vi "Re_run_Gnuplot.vi"(0 "Plot folder (dialog if empty)":path) -> ()   [LabVIEW 2014]
panel:
  in  "Data file":string
  in  "stop":bool
  in  "OK Button":bool
  in  "Gnuplot script file":string
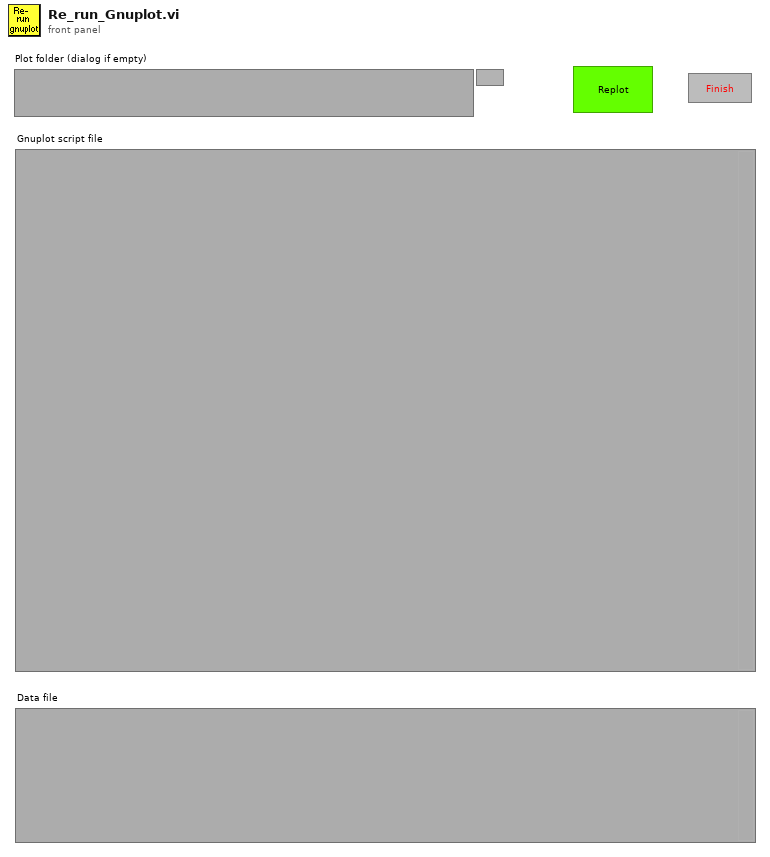
[diagram p1: front panel]
types:
  T1 = enum32{"existing file", "new file", "new or existing file", "existing dir", "new dir", "new or existing dir", "existing file (use LLBs)", "new file (use LLBs)", "new or existing file (use LLBs)", "new or existing file or directory (use LLBs)"}
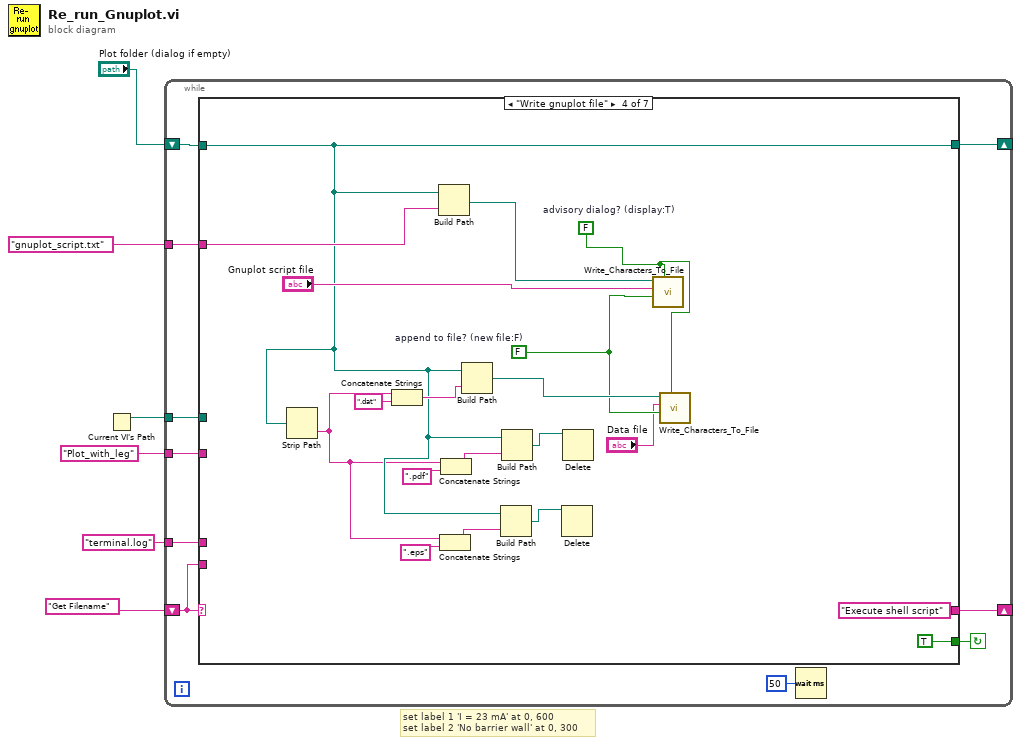
[diagram p0: block diagram]
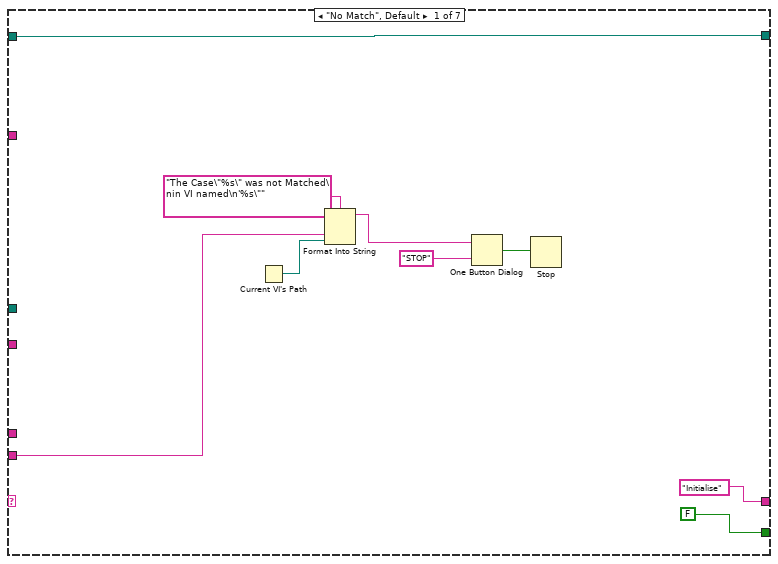
[diagram p2: hidden frame]
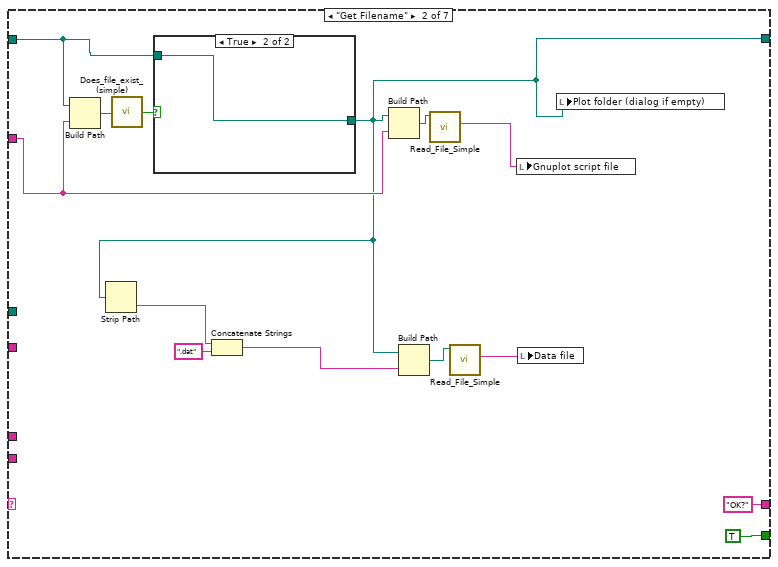
[diagram p3: hidden frame]
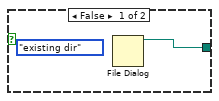
[diagram p4: hidden frame]
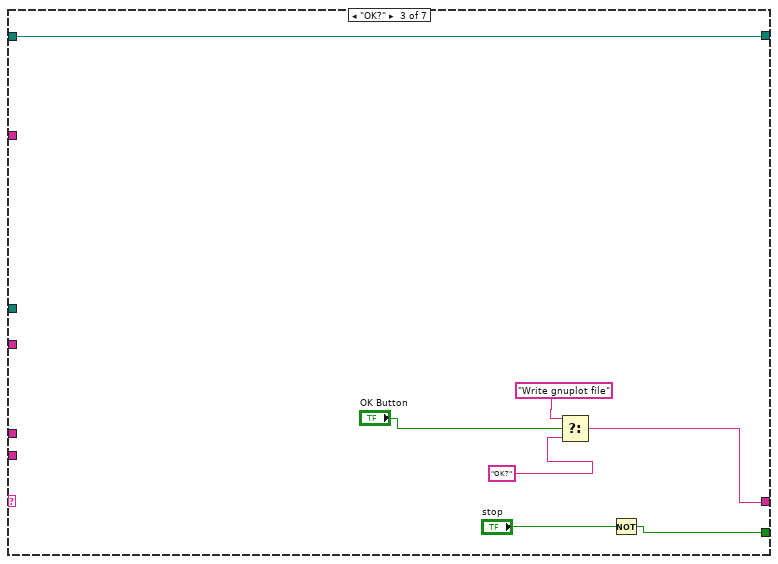
[diagram p5: hidden frame]
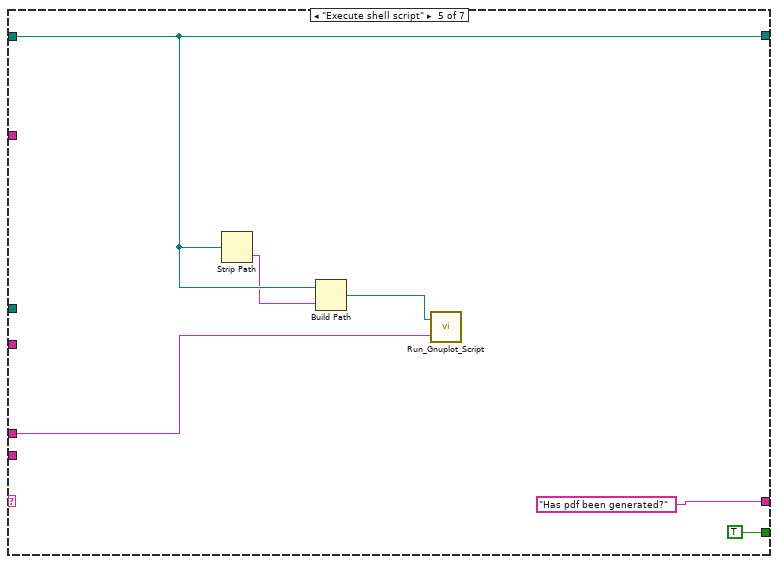
[diagram p6: hidden frame]
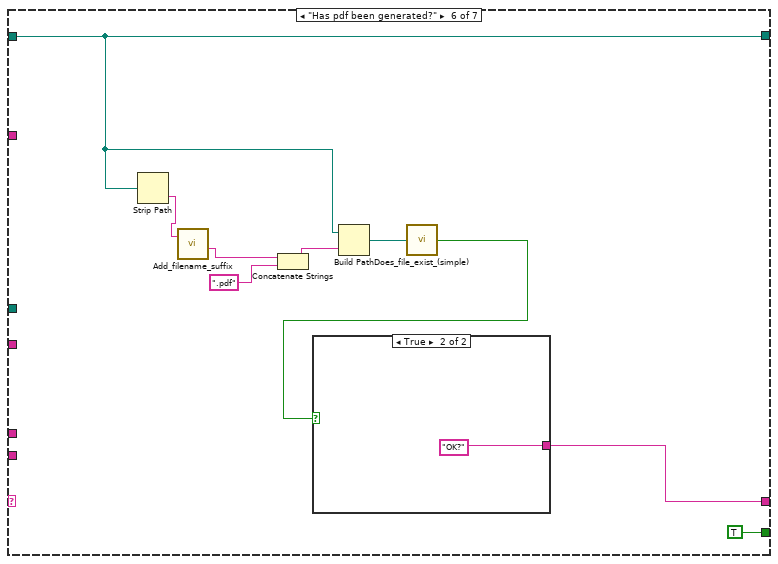
[diagram p7: hidden frame]
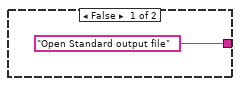
[diagram p8: hidden frame]
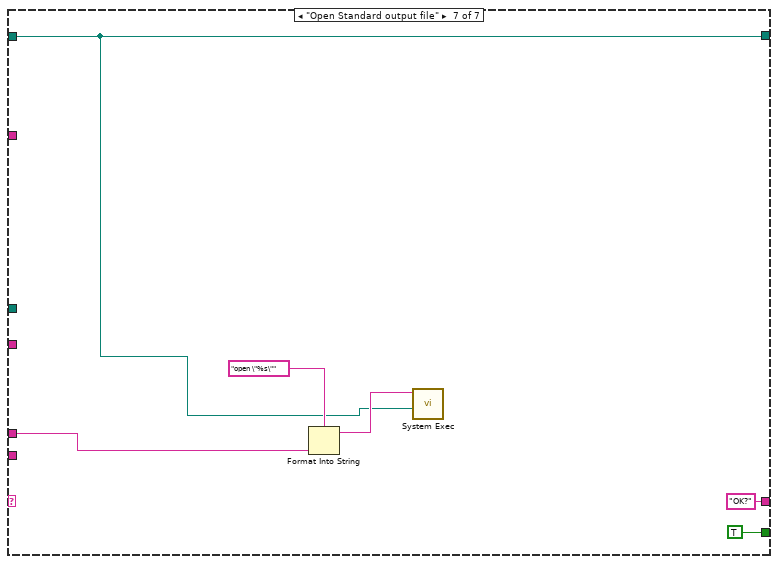
[diagram p9: hidden frame]
diagram:
  # "set label 1 'I = 23 mA' at 0, 600\nset label 2 'No barrier wall' at 0, 300"
  n1 = Current VI's Path() -> (path=w5:path)
  n2 = while {
    shift-left: "Get Filename" -> [w14]
    shift-right: [w15] -> _
    tunnel: w5 -> [w13]
    shift-right: [w12] -> _
    shift-left: "Plot folder (dialog if empty)" -> [w11]
    tunnel: "Plot_with_leg" ("name or relative path") -> [w10]
    tunnel: "terminal.log" -> [w9]
    tunnel: "gnuplot_script.txt" -> [w8]
    stop <- w16 continue-if-true
    n3 = case shown="\"Write gnuplot file\"" w14 {
      tunnel: [FALSE TRUE ("Top Level") w42 TRUE ("Top Level") TRUE ("Top Level") TRUE ("Top Level") TRUE ("Top Level")] -> w16
      tunnel: ["Initialise" "OK?" ("t") w48 "Execute shell script" ("t") "Has pdf been generated?" ("t") w79 "OK?" ("t")] -> w15
      tunnel: w14 -> [w20 _ _ _ _ _ _]
      tunnel: w13 -> [_ _ _ _ _ _ _]
      tunnel: [w17 w31 w45 w50 w70 w74 w85] -> w12
      tunnel: w11 -> [w17 w35 w45 w50 w70 w74 w85]
      tunnel: w10 -> [_ _ _ _ _ _ _]
      tunnel: w9 -> [_ _ _ _ w71 _ w87]
      tunnel: w8 -> [_ w34 _ w63 _ _ _]
      frame "No Match", Default {
        n4 = Current VI's Path() -> (path=w19:path)
        n5 = Format Into String(format string="The Case\"%s\" was not Matched\nin VI named\n'%s\"" ("Format String"), w20, w19) -> (resulting string=w23:string)  [unwired: 2 in, 1 out]
        n6 = One Button Dialog(message=w23, button name ("OK")="STOP") -> (true=w21:bool)
        n7 = Stop(stop? (T)=w21) -> ()
      }
      frame "Get Filename" {
        n8 = Build Path(base path=w35, name or relative path=w34) -> (appended path=w33:path)
        n9 = call "Does_file_exist_(simple).vi"("Pathname"=w33) -> ("exists?"=w32:bool)
        n10 = case shown="True" w32 {
          tunnel: [w40 w41] -> w31
          tunnel: w35 -> [_ w41]
          frame False {
            (unwired) T1."existing dir" ("select mode (2)")
            n11 = File Dialog() -> (3:w40:path)  [unwired: 1 in, 9 out]
          }
          frame True {
          }
        }
        n12 = Strip Path(path=w31) -> (name=w30:string)  [unwired: 1 out]
        n13 = Concatenate Strings(w30, ".dat" ("string")) -> (w28:string)
        n14 = Build Path(base path=w31, name or relative path=w34) -> (appended path=w36:path)
        n15 = Build Path(base path=w31, name or relative path=w28) -> (appended path=w27:path)
        n16 = call "Read_File_Simple.vi"("Filename"=w36) -> ("string"=w38:string)  [unwired: 2 in, 7 out]
        n17 = call "Read_File_Simple.vi"("Filename"=w27) -> ("string"=w26:string)  [unwired: 2 in, 7 out]
        n18 = local write "Gnuplot script file"(w38) -> ()
        n19 = local write "Data file"(w26) -> ()
        n20 = local write "Plot folder (dialog if empty)"(w31) -> ()
      }
      frame "OK?" {
        n21 = Select(t="Write gnuplot file", s="OK Button", f="OK?") -> (s? t:f=w48:string)
        n22 = Not(x="stop") -> (.not. x?=w42:bool)
      }
      frame "Write gnuplot file" {
        w59 = FALSE  # append to file? (new file:F)
        w58 = FALSE  # advisory dialog? (display:T)
        n23 = Strip Path(path=w50) -> (name=w49:string)  [unwired: 1 out]
        n24 = Concatenate Strings(w49, ".dat" ("string")) -> (w61:string)
        n25 = Build Path(base path=w50, name or relative path=w63) -> (appended path=w67:path)
        n26 = Concatenate Strings(w49, ".eps" ("string")) -> (w51:string)
        n27 = Concatenate Strings(w49, ".pdf" ("string")) -> (w56:string)
        n28 = Build Path(base path=w50, name or relative path=w61) -> (appended path=w60:path)
        n29 = Build Path(base path=w50, name or relative path=w51) -> (appended path=w53:path)
        n30 = Build Path(base path=w50, name or relative path=w56) -> (appended path=w54:path)
        n31 = Delete(path (use dialog)=w53) -> ()  [unwired: 1 in, 6 out]
        n32 = Delete(path (use dialog)=w54) -> ()  [unwired: 1 in, 6 out]
        n33 = call "Write_Characters_To_File.vi"("file path (dialog if empty)"=w67, "advisory dialog? (display:T)"=w58, "character string"="Gnuplot script file", "append to file? (new file:F)"=w59) -> ()  [unwired: 1 in, 4 out]
        n34 = call "Write_Characters_To_File.vi"("file path (dialog if empty)"=w60, "advisory dialog? (display:T)"=w58, "character string"="Data file", "append to file? (new file:F)"=w59) -> ()  [unwired: 1 in, 4 out]
      }
      frame "Execute shell script" {
        n35 = Strip Path(path=w70) -> (name=w69:string)  [unwired: 1 out]
        n36 = Build Path(base path=w70, name or relative path=w69) -> (appended path=w68:path)
        n37 = call "Run_Gnuplot_Script.vi"("logfileName"=w71, "workingDirectory"=w68) -> ()
      }
      frame "Has pdf been generated?" {
        n38 = Strip Path(path=w74) -> (name=w76:string)  [unwired: 1 out]
        n39 = call "Add_filename_suffix.vi"("Filename"=w76) -> ("Base name"=w75:string)  [unwired: 1 in, 3 out]
        n40 = Concatenate Strings(w75, ".pdf" ("string")) -> (w82:string)
        n41 = Build Path(base path=w74, name or relative path=w82) -> (appended path=w80:path)
        n42 = call "Does_file_exist_(simple).vi"("Pathname"=w80) -> ("exists?"=w78:bool)
        n43 = case shown="True" w78 {
          tunnel: ["Open Standard output file" ("f") "OK?" ("t")] -> w79
          frame False {
          }
          frame True {
          }
        }
      }
      frame "Open Standard output file" {
        n44 = Format Into String(format string="open \"%s\"", w87) -> (resulting string=w86:string)  [unwired: 2 in, 1 out]
        n45 = call <vilib>:"System Exec.vi"("working directory"=w85, "command line"=w86) -> ()  [unwired: 4 in, 6 out]
      }
    }
    n46 = Wait (ms)(milliseconds to wait=u32 50) -> ()  [unwired: 1 out]
  }
